vi "aryth_block.vi"(2 "C":T1, 3 "S-1":bool, 4 "B":bool, 5 "A":bool) -> (0 "R":bool, 1 "S1":bool)   [LabVIEW 2013]
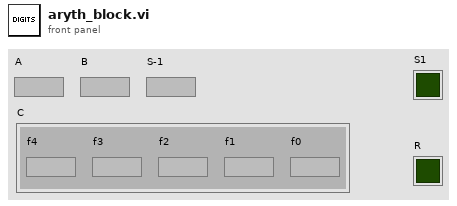
[diagram p1: front panel]
types:
  T1 = cluster{"f4":bool, "f3":bool, "f2":bool, "f1":bool, "f0":bool}
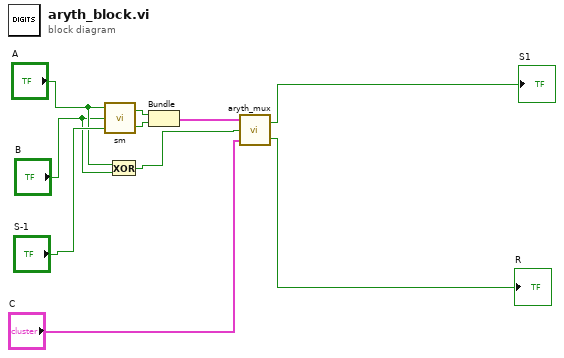
[diagram p0: block diagram]
diagram:
  n1 = call "sm.vi"("c"="S-1", "b"="B", "a"="A") -> ("C"=w6:bool, "S"=w7:bool)
  n2 = Exclusive Or(1:"B", 2:"A") -> (0:w4:bool)
  n3 = Bundle("S"=w7, "C"=w6) -> (w5:cluster{"S":bool, "C":bool})  [unwired: 1 in]
  n4 = call "aryth_mux.vi"("C"="C", "A-B"=w4, "A+B"=w5) -> ("R"=→"R":bool, "S1"=→"S1":bool)
